vi "populate_settings_list.vi"(8 "error in (no error)":errorcluster, 9 "available settings":T1[](array[typedef]), 10 "list ref":refnum<vi>, 11 "GenericPlugin in":refnum<class "GenericComponent.lvclass">) -> (0 "error out":errorcluster, 3 "GenericPlugin out":refnum<class "GenericComponent.lvclass">)   [LabVIEW 2010, in "GenericComponent.lvclass"]
uses:
  GenericComponent.lvclass
  clusters/settings_specification_cluster.ctl
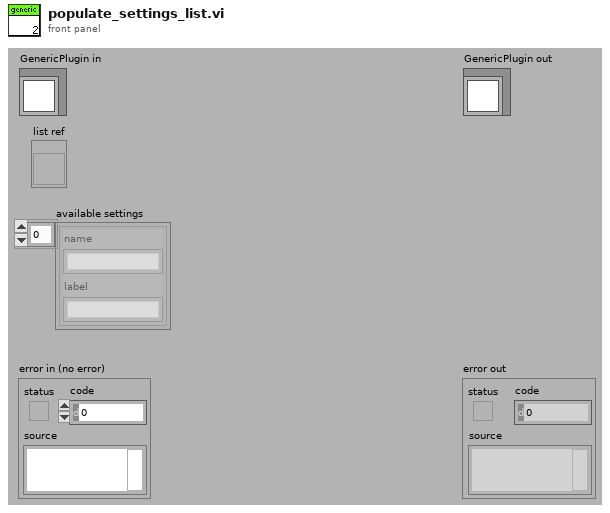
[diagram p1: front panel]
types:
  T1 = typedef "settings_specification_cluster.ctl" = cluster{"name":string, "label":string}
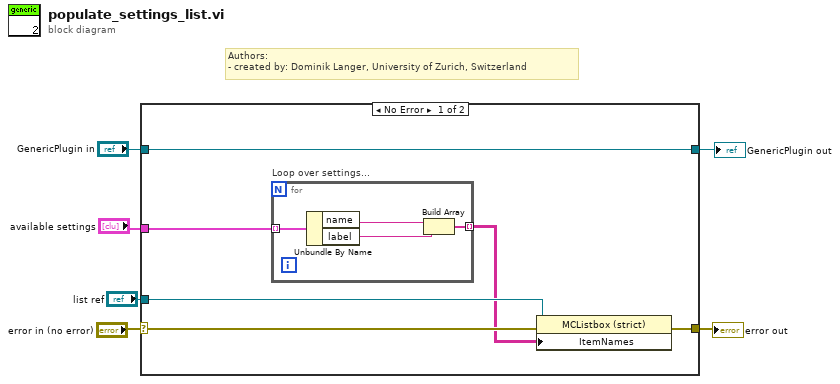
[diagram p0: block diagram]
diagram:
  # "Authors: \n- created by: Dominik Langer, University of Zurich, Switzerland"
  n1 = case shown="No Error" "error in (no error)" {
    selector: "error in (no error)" -> [w12 w18]
    tunnel: [w11 w18] -> w3
    tunnel: [w8 w17] -> w6
    tunnel: "GenericPlugin in" -> [w8 w17]
    tunnel: "list ref" -> [w10 _]
    tunnel: "available settings" -> [w7 _]
    frame No Error {
      n2 = for "Loop over settings..." {
        tunnel: w7 -> [w16] mode=indexing
        tunnel: [w14] -> w9 mode=indexing
        n3 = Unbundle By Name(w16) -> ("name"=w13:string, "label"=w15:string)
        n4 = Build Array(w13, w15) -> (w14:string[])
      }
      n5 = property on="Property Node" class="MCListbox (strict)"(reference=w10, error in=w12, "ItemNames"=w9) -> (error out=w11:errorcluster)  [unwired: 1 out]
    }
    frame Error {
    }
  }
  "error out" <- w3
  "GenericPlugin out" <- w6
